vi "setLogicOutChannel.vi"(7 "outputTypeStr":string, 8 "error in (no error)":errorcluster, 9 "polarityStr":string, 11 "pHandle":u32) -> (0 "error out":errorcluster, 3 "return type":i32)   [LabVIEW 2011, in "sbgLabView.lvlib"]
uses:
  sbgLabView.lvlib
  sbgMatLab.dll
panel:
  in  "duration":u8
  in  "channel":u8
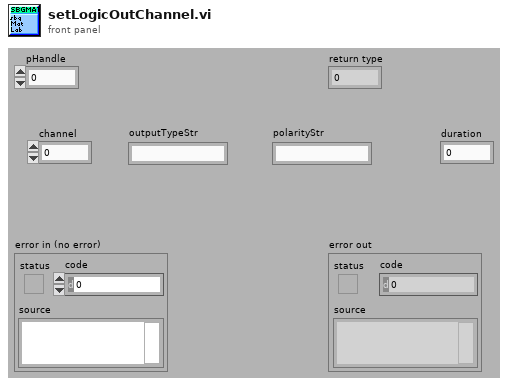
[diagram p1: front panel]
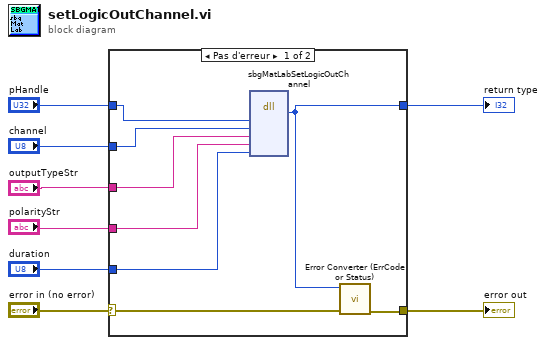
[diagram p0: block diagram]
diagram:
  n1 = case shown="Pas d'erreur" "error in (no error)" {
    selector: "error in (no error)" -> [w14 w17]
    tunnel: [w13 w17] -> w7
    tunnel: [w16 _] -> w6
    tunnel: "pHandle" -> [w15 _]
    tunnel: "outputTypeStr" -> [w11 _]
    tunnel: "polarityStr" -> [w10 _]
    tunnel: "channel" -> [w12 _]
    tunnel: "duration" -> [w9 _]
    frame No Error {
      n2 = dll-call lib="C:/SBG-Systems/remote/projects/software/projects/labviewExample/sbgLabView/sbgMatLab.*" fn="sbgMatLabSetLogicOutChannel" ("sbgMatLab.dll:sbgMatLabSetGpsOptions")("pHandle"=w15, "channel"=w12, "outputTypeStr"=w11, "polarityStr"=w10, "duration"=w9) -> ("return type"=w16:i32)  [unwired: 8 in, 2 out]
      n3 = call "Error Converter (ErrCode or Status).vi"("error in (no error)"=w14, "error code"=w16) -> ("error out"=w13:errorcluster)  [unwired: 9 in]
    }
    frame Error {
    }
  }
  "return type" <- w6
  "error out" <- w7
